vi "calculate_alkalinity.vi"(0 "Run Settings":T1, 1 "Alkalinity Calculation Functions":T4, 2 "Titration Points":T3, 3 "HCl Concentration":dbl, 4 "HCl Temp (uncorr)":dbl) -> (5 "Probe 1 Results":T2, 6 "Probe 2 Results":T2)   [LabVIEW 2010]
uses:
  <vilib>/gmath/NI_Gmath.lvlib
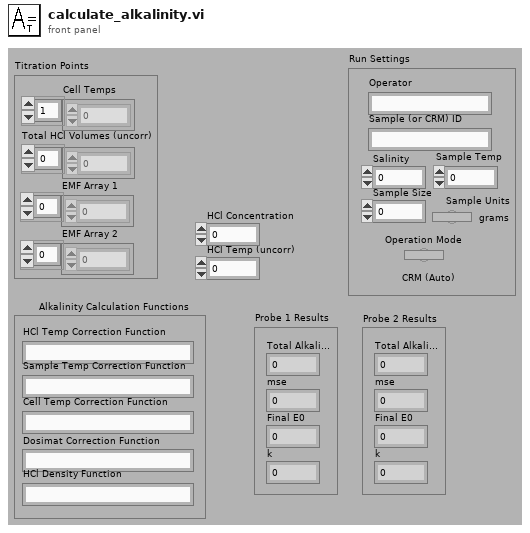
[diagram p1: front panel]
types:
  T1 = cluster{"Operator":string, "Sample (or CRM) ID":string, "Sample Temp":dbl, "Salinity":dbl, "Sample Units":bool, "Sample Size":dbl, "Operation Mode":bool}
  T2 = cluster{"Total Alkalinity":dbl, "mse":dbl, "Final E0":dbl, "k":dbl}
  T3 = cluster{"Cell Temps":dbl[], "Total HCl Volumes (uncorr)":dbl[], "EMF Array 1":dbl[], "EMF Array 2":dbl[]}
  T4 = cluster{"HCl Temp Correction Function":string, "Sample Temp Correction Function":string, "Dosimat Correction Function":string, "Cell Temp Correction Function":string, "HCl Density Function":string}
  T5 = cluster{"FitAlk":dbl, "mse":dbl, "FitE0":dbl, "k":dbl}
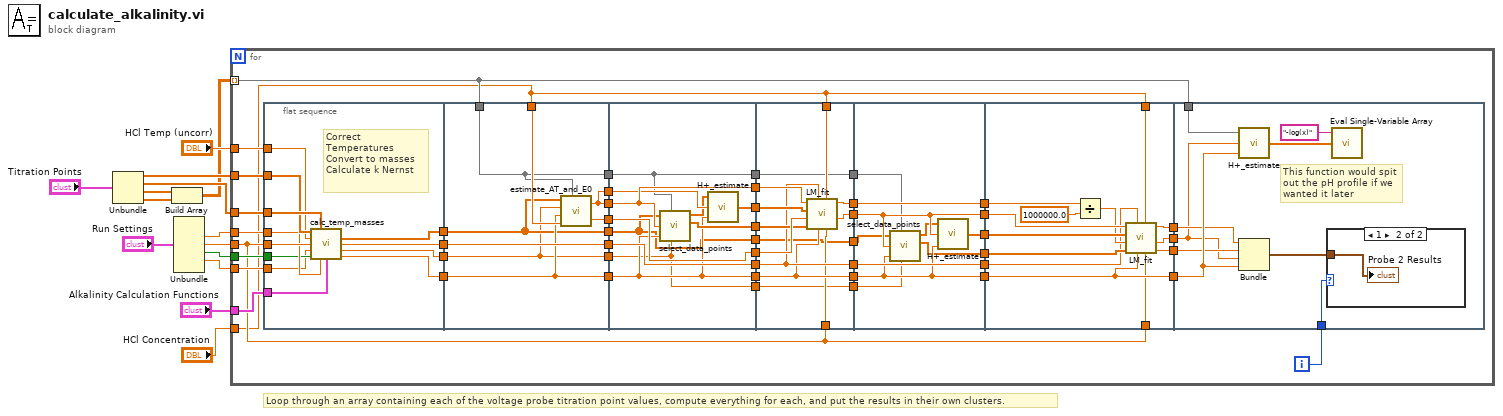
[diagram p0: block diagram]
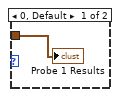
[diagram p2: hidden frame]
diagram:
  # "Loop through an array containing each of the voltage probe titration point values, compute everything for each, and put the results in their own clusters."
  n1 = Unbundle("Titration Points") -> ("Cell Temps"=w10:dbl[], "Total HCl Volumes (uncorr)"=w9:dbl[], "EMF Array 1"=w8:dbl[], "EMF Array 2"=w7:dbl[])
  n2 = Build Array(w8, w7) -> (w6:dbl[][])
  n3 = Unbundle("Run Settings") -> ("Sample Temp"=w4:dbl, "Salinity"=w3:dbl, "Sample Units"=w2:bool, "Sample Size"=w1:dbl)  [unwired: 3 out]
  n4 = for {
    tunnel: "Alkalinity Calculation Functions" -> [w31]
    tunnel: "HCl Temp (uncorr)" -> [w30]
    tunnel: "HCl Concentration" -> [w21]
    tunnel: w10 -> [w29]
    tunnel: w9 -> [w28]
    tunnel: w3 -> [w22]
    tunnel: w4 -> [w27]
    tunnel: w2 -> [w26]
    tunnel: w1 -> [w25]
    tunnel: w6 -> [w24] mode=indexing
    i -> [w23]
    n5 = flat-sequence {
      tunnel: [w75] -> w63
      tunnel: w31 -> [w68]
      tunnel: w28 -> [w74]
      tunnel: w29 -> [w73]
      tunnel: w30 -> [w72]
      tunnel: [w71] -> w62
      tunnel: [w64] -> w61
      tunnel: [w70] -> w60
      tunnel: w22 -> [w69]
      tunnel: w27 -> [w67]
      tunnel: w26 -> [w66]
      tunnel: w25 -> [w65]
      tunnel: [w83] -> w59
      tunnel: [w82] -> w58
      tunnel: [w76] -> w57
      tunnel: w63 -> [w83]
      tunnel: w21 -> [w81]
      tunnel: w62 -> [w80]
      tunnel: w61 -> [w77]
      tunnel: w60 -> [w79]
      tunnel: w24 -> [w78]
      tunnel: [w80] -> w56
      tunnel: [w79] -> w55
      tunnel: [w78] -> w54
      tunnel: [w77] -> w53
      tunnel: [w76] -> w52
      tunnel: w59 -> [w94]
      tunnel: [w94] -> w51
      tunnel: w58 -> [w93]
      tunnel: [w93] -> w50
      tunnel: w57 -> [w91]
      tunnel: [w91] -> w49
      tunnel: [w88] -> w48
      tunnel: [w92] -> w47
      tunnel: w56 -> [w87]
      tunnel: w55 -> [w86]
      tunnel: w54 -> [w85]
      tunnel: w53 -> [w84]
      tunnel: w52 -> [w90]
      tunnel: [w87] -> w46
      tunnel: [w86] -> w19
      tunnel: [w85] -> w18
      tunnel: [w84] -> w15
      tunnel: w51 -> [w101]
      tunnel: w50 -> [w106]
      tunnel: w49 -> [w107]
      tunnel: [w105] -> w45
      tunnel: [w104] -> w44
      tunnel: [w101] -> w43
      tunnel: w48 -> [w103]
      tunnel: w47 -> [w102]
      tunnel: w46 -> [w100]
      tunnel: [w100] -> w42
      tunnel: w21 -> [w99]
      tunnel: w22 -> [w98]
      tunnel: [w97] -> w20
      tunnel: w19 -> [w97]
      tunnel: w18 -> [w96]
      tunnel: [w96] -> w17
      tunnel: [w95] -> w16
      tunnel: w15 -> [w95]
      tunnel: w45 -> [w116]
      tunnel: [w116] -> w41
      tunnel: w44 -> [w114]
      tunnel: [w114] -> w40
      tunnel: [w109] -> w39
      tunnel: w43 -> [w117]
      tunnel: [w117] -> w38
      tunnel: [w115] -> w37
      tunnel: w42 -> [w113]
      tunnel: [w113] -> w36
      tunnel: w20 -> [w112]
      tunnel: w17 -> [w111]
      tunnel: w16 -> [w110]
      tunnel: w41 -> [w125]
      tunnel: w40 -> [w130]
      tunnel: w39 -> [w129]
      tunnel: w38 -> [w122]
      tunnel: [w128] -> w35
      tunnel: [w127] -> w34
      tunnel: w37 -> [w126]
      tunnel: w36 -> [w120]
      tunnel: [w121] -> w33
      tunnel: [w120] -> w32
      tunnel: w22 -> [w119]
      tunnel: w21 -> [w118]
      tunnel: w35 -> [w133]
      tunnel: w34 -> [w134]
      tunnel: w24 -> [w137]
      tunnel: w33 -> [w132]
      tunnel: w32 -> [w135]
      tunnel: w23 -> [w136]
      frame #0 {
        # "Correct Temperatures\nConvert to masses\nCalculate k Nernst"
        n6 = call "calc_temp_masses.vi"("Cell Temps (uncorr)"=w73, "Total HCl Volumes (uncorr)"=w74, "HCl Temp (burret)"=w72, "Salinity"=w69, "Sample Size"=w65, "Sample Units"=w66, "Sample Temp (uncorr)"=w67, "Alkalinity Calculation Functions"=w68) -> ("Total HCl masses"=w70:dbl[], "Corrected Cell Temperature Mean"=w75:dbl, "Sample Mass"=w64:dbl, "k"=w71:dbl)  [unwired: 3 in, 1 out]
      }
      frame #1 {
        n7 = call "estimate_AT_and_E0.vi"("EMFs"=w78, "HCl Concentration"=w81, "k"=w80, "Sample Mass"=w77, "Total HCl masses"=w79) -> ("AT Estimate"=w82:dbl, "E0 Estimate"=w76:dbl)  [unwired: 1 in]
      }
      frame #2 {
        n8 = call "select_data_points.vi"("Total HCl masses"=w86, "EMFs"=w85, "E0"=w91, "k"=w87, "Sample Mass"=w84) -> ("EMF Array (pH3-3.5)"=w89:dbl[], "m/m0 Array"=w92:dbl[])  [unwired: 2 out]
        n9 = call "H+_estimate.vi"("k"=w87, "EO Estimate"=w90, "EMFs (pH3-3.5)"=w89) -> ("H+ Estimate"=w88:dbl[])
      }
      frame #3 {
        n10 = call "LM_fit.vi"("Salinity"=w98, "HCl Concentration"=w99, "k"=w100, "Corrected Cell Temperature Mean"=w101, "m/m0"=w102, "TA estimate"=w106, "H+ estimate"=w103, "E0 estimate"=w107) -> ("FitE0"=w104:dbl, "FitAlk"=w105:dbl)  [unwired: 1 in, 1 out]
      }
      frame #4 {
        n11 = call "select_data_points.vi"("Total HCl masses"=w112, "EMFs"=w111, "E0"=w114, "k"=w113, "Sample Mass"=w110) -> ("EMF Array (pH3-3.5)"=w108:dbl[], "m/m0 Array"=w109:dbl[])  [unwired: 2 out]
        n12 = call "H+_estimate.vi"("k"=w113, "EO Estimate"=w114, "EMFs (pH3-3.5)"=w108) -> ("H+ Estimate"=w115:dbl[])
      }
      frame #5 {
        n13 = Divide(x=w125, y=1000000.0) -> (x/y=w123:dbl)
        n14 = call "LM_fit.vi"("Salinity"=w119, "HCl Concentration"=w118, "k"=w120, "Corrected Cell Temperature Mean"=w122, "m/m0"=w129, "TA estimate"=w123, "H+ estimate"=w126, "E0 estimate"=w130) -> ("mse"=w127:dbl, "FitE0"=w121:dbl, "FitAlk"=w128:dbl)  [unwired: 1 in]
      }
      frame #6 {
        # "This function would spit out the pH profile if we wanted it later"
        n15 = call "H+_estimate.vi"("k"=w135, "EO Estimate"=w132, "EMFs (pH3-3.5)"=w137) -> ("H+ Estimate"=w138:dbl[])
        n16 = Bundle("FitAlk"=w133, "mse"=w134, "FitE0"=w132, "k"=w135) -> (w131:T5)  [unwired: 1 in]
        n17 = case shown="1" w136 {
          tunnel: w131 -> [w140 w141]
          frame 0, Default {
            "Probe 1 Results" <- w140
          }
          frame 1 {
            "Probe 2 Results" <- w141
          }
        }
        n18 = call <vilib>:"Eval Single-Variable Array.vi"("X Values"=w138, "formula"="-log(x)") -> ()  [unwired: 1 in, 2 out]
      }
    }
  }
